vi "setLetterSpacing.vi"(8 "Error In":errorcluster, 9 "spacing":dbl, 10 "type":T1 items=["PercentageSpacing", "AbsoluteSpacing"], 11 "QFont In":refnum<class "QFont.lvclass">) -> (0 "Error Out":errorcluster, 3 "QFont Out":refnum<class "QFont.lvclass">)   [LabVIEW 2014, in "QFont.lvclass"]
doc: "LabVIEW-specific documentation is not yet available. See <b>http://doc.qt.io/qt-5/QFont.html#setLetterSpacing</b>"
uses:
  QFont.lvclass
  SpacingType.ctl
  LQ Core/LQSerialData/LQSerialData.lvclass/LQSerialData.ctl
  LQ Core/LQ Core.lvlib
  LQ Core/LQSerialData/LQSerialData.lvclass
panel:
  # "Copyright (c) 2016 Sze Howe Koh\n\nThis Source Code Form is subject to the terms of the Mozilla Public\nLicense, v. 2.0. If a copy of the MPL was not distributed with this\nfile, You can obtain one at http://mozilla.org/MPL/2.0/."
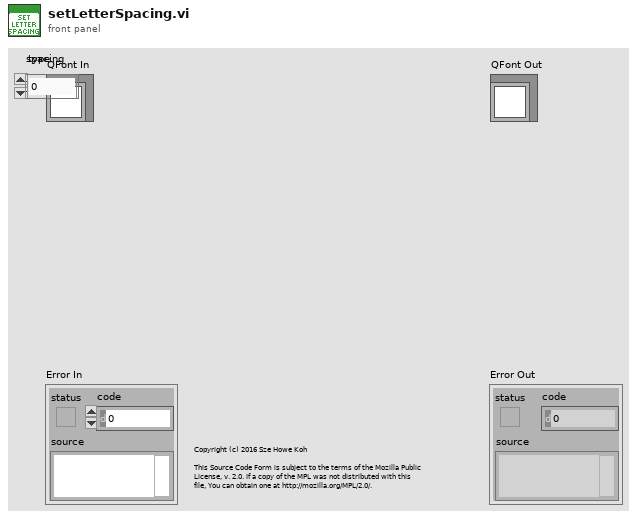
[diagram p1: front panel]
types:
  T1 = typedef "QFont.lvclass/SpacingType.ctl" = i32
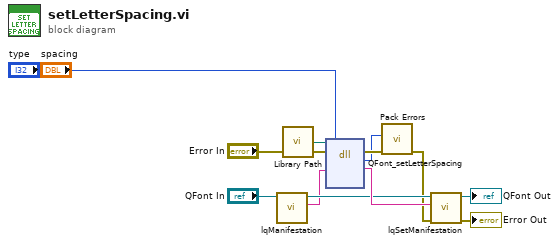
[diagram p0: block diagram]
diagram:
  n1 = call "lqManifestation.vi"("LQSerialData in"="QFont In") -> ("Manifestation"=w8:string, "LQSerialData out"=w9:refnum<class "QFont.lvclass">)  [unwired: 9 in]
  n2 = call "Library Path.vi"() -> ("Library Path"=w7:path)
  n3 = dll-call lib="?" fn="QFont_setLetterSpacing"(path in=w7, error in="Error In", "_instance"=w8, "type"="type", "spacing"="spacing") -> (error out=w6:errorcluster, w5:i32, "_instance"=w11:string)  [unwired: 3 in, 1 out]
  n4 = call "Pack Errors.vi"("Error In"=w6, "Error Code"=w5) -> ("Error Out"=w4:errorcluster)  [unwired: 9 in]
  n5 = call "lqSetManifestation.vi"("Error In"=w4, "Manifestation"=w11, "LQSerialData in"=w9) -> ("Error Out"=→"Error Out":errorcluster, "LQSerialData out"=→"QFont Out":refnum<class "QFont.lvclass">)  [unwired: 7 in]
